vi "Init VI Module.vi"(8 "error in":errorcluster, 11 "Module Admin in":refnum<class "lib_QMH_Module_Admin.lvclass">) -> (0 "error out":errorcluster, 3 "Module Admin out":refnum<class "lib_QMH_Module_Admin.lvclass">)   [LabVIEW 2018]
uses:
  Module Admin_class/lib_QMH_Module_Admin.lvclass
  Module Admin_class/lib_QMH_Module_Admin.lvclass/lib_QMH_Module_Admin.ctl
  Module Admin_class/lib_QMH_Get Show Diagram on Init.vi
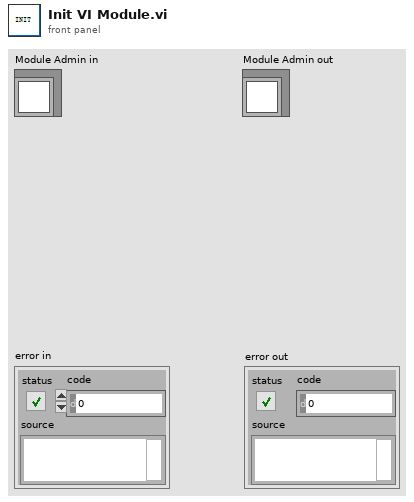
[diagram p1: front panel]
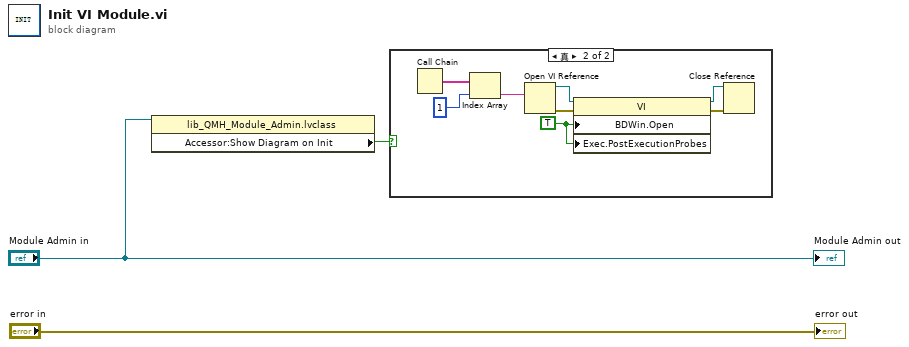
[diagram p0: block diagram]
diagram:
  n1 = property class="lib_QMH_Module_Admin.lvclass"(reference="Module Admin in") -> ("Accessor:Show Diagram on Init"=w3:bool)  [unwired: 1 in, 2 out]
  n2 = case shown="真" w3 {
    frame False {
    }
    frame True {
      w7 = TRUE ("Block Diagram Window:Open")
      n3 = Call Chain() -> (call chain=w11:string[])
      n4 = Index Array(array=w11, index=1) -> (element=w4:string)
      n5 = Open VI Reference(vi path=w4) -> (vi reference=w8:refnum<vi>, error out=w9:errorcluster)  [unwired: 5 in]
      n6 = property class="VI"(reference=w8, error in=w9, "BDWin.Open"=w7, "Exec.PostExecutionProbes"=w7) -> (reference out=w5:refnum<vi>, error out=w6:errorcluster)
      n7 = Close Reference(reference=w5, error in (no error)=w6) -> ()  [unwired: 1 out]
    }
  }
  "error out" <- "error in"
  "Module Admin out" <- "Module Admin in"
